vi "ATI-mini40.vi"() -> ()   [LabVIEW 2018]
uses:
  <vilib>/Platform/TimedLoop/XDataNode/timing_clust.ctl
  <vilib>/Platform/TimedLoop/XDataNode/nitl_modes.ctl
  <vilib>/Platform/TimedLoop/XDataNode/wakeup.ctl
  <vilib>/Platform/TimedLoop/XDataNode/loadnilvce.vi
  <vilib>/Platform/TimedLoop/XDataNode/XDataNode.xnode
  <vilib>/Platform/TimedLoop/XDataNode/XDNodeRunTimeDep.lvlib
panel:
  in  "Filter":u16(ring)=3 items=["Filter1", "Filter2", "Filter3", "Filter4"]
  in  "Calibration":u16(ring) items=["SI-20-1", "SI-40-2"]
  in  "Zeroing":bool
  out "Error":bool
  out "Mini-40":T1 {"Fx" format="%.6f"; "Fy" format="%.6f"; "Fz" format="%.6f"; "Tx" format="%.6f"; "Ty" format="%.6f"; "Tz" format="%.6f"}
  in  "Stop":bool
  out "Status":bool[](array[boolean])
  out "Ctrl1":bool[](array[boolean])
  # "Reset"
  # "Filter1"
  # "Filter2"
  # "Filter3"
  # "Filter4"
  # "Calib1"
  # "Calib2"
  # "Calib3"
  # "Calib4"
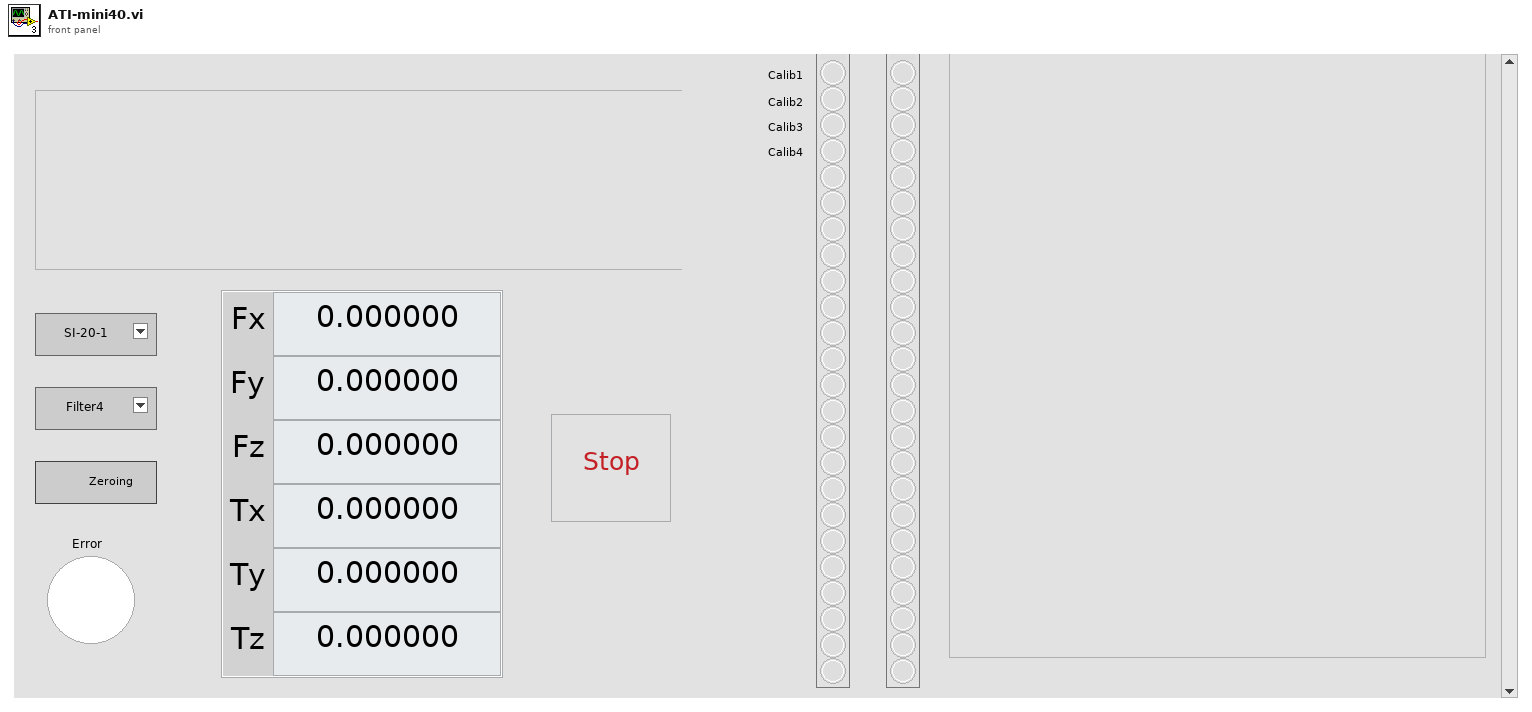
[diagram p1: front panel]
types:
  T1 = cluster{"Fx":dbl, "Fy":dbl, "Fz":dbl, "Tx":dbl, "Ty":dbl, "Tz":dbl}
  T2 = typedef "XDNodeRunTimeDep.lvlib/timing_clust.ctl" = cluster{"Expected End [f-1]":u64, "Actual End [f-1]":u64, "Finished Late? [f-1]":bool, "Expected End [i-1]":u64, "Actual End [i-1]":u64, "Finished Late? [i-1]":bool, "Expected Start [i]":u64, "Actual Start [i]":u64, "Expected Start [f]":u64, "Actual Start [f]":u64, "Source Name":string, "Structure Name":string, "Period":i64, "Deadline":i64, "Offset":i64, "Start":i64, "Priority":i32, "Timeout":i32, "Mode":T3, "Wakeup Reason":T4, "Error":errorcluster, "Source Type":string, "Secondary Source Type":string, "Global End Time":u64, "Global Start Time":u64, "Frame Duration":u64, "Iteration Duration":u64, "Assigned CPU":i32, "I/O Scan Engine Mode":u32}
  T3 = typedef "XDNodeRunTimeDep.lvlib/nitl_modes.ctl" = enum32{"No Change", "Process missed periods, maintain original phase", "Discard missed periods, maintain original phase", "Process missed periods, ignore original phase", "Discard missed periods, ignore original phase"}
  T4 = typedef "XDNodeRunTimeDep.lvlib/wakeup.ctl" = enum32{"Normal", "Aborted", "Asynchronous wakeup", "Timing source error", "Timed loop error", "Timeout"}
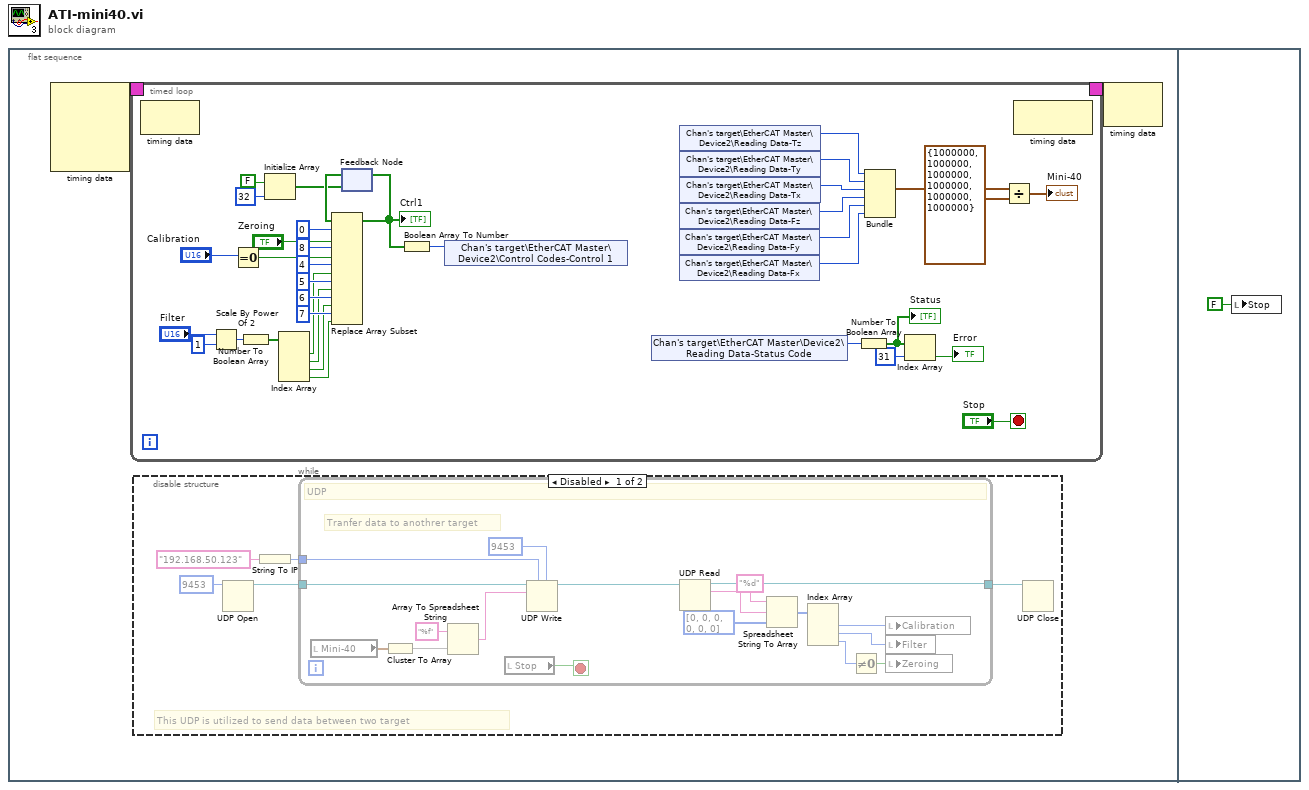
[diagram p0: block diagram]
diagram:
  n1 = flat-sequence {
    frame #0 {
      n2 = node-c288() -> (w2:T2)  [unwired: 4 in]
      n3 = timed-loop {
        timing: w2 -> [_]
        timing-out: [_] -> w1
        stop <- "Stop" stop-if-true
        n4 = node-c288() -> ()  [unwired: 1 in, 1 out]
        n5 = Scale By Power Of 2(n="Filter", x=u8 1) -> (x*2^n=w40:u8)
        n6 = Equal To 0?(x="Calibration") -> (x = 0?=w54:bool)
        n7 = Number To Boolean Array(number=w40) -> (Boolean array=w39:bool[])
        n8 = Initialize Array(FALSE, 32 ("dimension size")) -> (w49:bool[])
        n9 = Index Array(array=w39) -> (element #1=w38:bool, element #2=w37:bool, element #3=w36:bool, element #4=w35:bool)  [unwired: 4 in]
        n10 = feedback #1(w49) -> (w56:bool[])
        n11 = Replace Array Subset(array=w56, new element #1="Zeroing", index #1=0 ("index"), new element #2=w54, index #2=8 ("index"), new element #3=w38, index #3=4 ("index"), new element #4=w37, index #4=5 ("index"), new element #5=w36, index #5=6 ("index"), new element #6=w35, index #6=7 ("index")) -> (w47:bool[])
        "Ctrl1" <- w47
        n12 = feedback-in #1(w47) -> ()
        n13 = Boolean Array To Number(Boolean array=w47) -> (number=w27:u32)
        n14 = shared-variable "Chan's target\\EtherCAT Master\\Device2\\Control Codes-Control 1"(w27) -> ()  [unwired: 1 in, 1 out]
        n15 = shared-variable "Chan's target\\EtherCAT Master\\Device2\\Reading Data-Status Code"() -> (w26:u32)  [unwired: 1 in, 1 out]
        n16 = shared-variable "Chan's target\\EtherCAT Master\\Device2\\Reading Data-Tz"() -> (w33:i32)  [unwired: 1 in, 1 out]
        n17 = shared-variable "Chan's target\\EtherCAT Master\\Device2\\Reading Data-Ty"() -> (w32:i32)  [unwired: 1 in, 1 out]
        n18 = shared-variable "Chan's target\\EtherCAT Master\\Device2\\Reading Data-Tx"() -> (w31:i32)  [unwired: 1 in, 1 out]
        n19 = shared-variable "Chan's target\\EtherCAT Master\\Device2\\Reading Data-Fz"() -> (w30:i32)  [unwired: 1 in, 1 out]
        n20 = shared-variable "Chan's target\\EtherCAT Master\\Device2\\Reading Data-Fy"() -> (w29:i32)  [unwired: 1 in, 1 out]
        n21 = shared-variable "Chan's target\\EtherCAT Master\\Device2\\Reading Data-Fx"() -> (w28:i32)  [unwired: 1 in, 1 out]
        n22 = Number To Boolean Array(number=w26) -> (Boolean array=w34:bool[])
        "Status" <- w34
        n23 = Bundle(w33, w32, w31, w30, w29, w28) -> (w61:cluster{i32, i32, i32, i32, i32, i32})  [unwired: 1 in]
        n24 = Index Array(array=w34, index=31) -> (element=→"Error":bool)
        n25 = Divide(x=w61, y=cluster{i32, i32, i32, i32, i32, i32} {1000000, 1000000, 1000000, 1000000, 1000000, 1000000}) -> (x/y=→"Mini-40":cluster{dbl, dbl, dbl, dbl, dbl, dbl})
        n26 = node-c288() -> ()  [unwired: 1 in, 1 out]
      }
      n27 = disable-structure shown="Disabled" {
        frame Disabled {
          # "This UDP is utilized to send data between two target"
          n28 = UDP Open(11:u16 9453 ("port")) -> (port=w7:refnum<k16>)  [unwired: 4 in, 2 out]
          n29 = String To IP(1:"192.168.50.123" ("name")) -> (0:w5:u32)
          n30 = while {
            tunnel: w7 -> [w25]
            tunnel: [w16] -> w6
            tunnel: w5 -> [w24]
            stop <- w21 stop-if-true
            # "Tranfer data to anothrer target"
            # "UDP"
            n31 = local read "Mini-40"() -> (w22:T1)
            n32 = Cluster To Array(cluster=w22) -> (array=w18:dbl[])
            n33 = Array To Spreadsheet String(array=w18, 3:"%f" ("format string")) -> (spreadsheet string=w19:string)  [unwired: 1 in]
            n34 = local read "Stop"() -> (w21:bool)
            n35 = UDP Write(address=w24, port or service name=u16 9453, connection ID=w25, data in=w19) -> (3:w17:refnum<k16>)  [unwired: 2 in, 1 out]
            n36 = UDP Read(connection ID=w17) -> (data out=w12:string, 3:w16:refnum<k16>)  [unwired: 3 in, 3 out]
            n37 = Spreadsheet String To Array(format string="%d", spreadsheet string=w12, array type (2D Dbl)=u16[] [0, 0, 0, 0, 0, 0]) -> (array=w13:u16[])  [unwired: 1 in]
            n38 = Index Array(array=w13) -> (element #1=w11:u16, element #2=w10:u16, element #3=w9:u16)  [unwired: 3 in]
            n39 = Not Equal To 0?(x=w9) -> (x != 0?=w8:bool)
            n40 = local write "Calibration"(w11) -> ()
            n41 = local write "Filter"(w10) -> ()
            n42 = local write "Zeroing"(w8) -> ()
          }
          n43 = UDP Close(connection ID=w6) -> ()  [unwired: 1 in, 2 out]
        }
        frame Enabled {
        }
      }
      n44 = node-c288(w1) -> ()  [unwired: 1 out]
    }
    frame #1 {
      n45 = local write "Stop"(FALSE ("Stop")) -> ()
    }
  }
